vi "SE Update Type.vi"(7 "Name":string, 8 "error in (no error)":errorcluster, 9 "Type":string, 10 "Child Refs":T1[](array[typedef]) format="%.0x", 11 "Type":T2) -> (0 "error out":errorcluster)   [LabVIEW 2015, in "RefMem DMA Custom Device.lvlib"]
uses:
  RefMem DMA Custom Device.lvlib
  Controls/Data Channel Type.ctl
  Program Files (x86)/National Instruments/LabVIEW 2015/vi.lib/NI Veristand/Custom Device API/Custom Device Item Ref.ctl
  Program Files (x86)/National Instruments/LabVIEW 2015/vi.lib/NI Veristand/Custom Device API/Custom Device Channel Type.ctl
  Program Files (x86)/National Instruments/LabVIEW 2015/vi.lib/NI Veristand/Custom Device API/Set Item Property (U16).vi
  Program Files (x86)/National Instruments/LabVIEW 2015/vi.lib/NI Veristand/Custom Device API/Custom Device API.lvlib
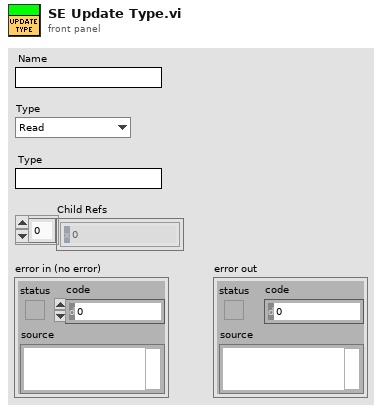
[diagram p1: front panel]
types:
  T1 = typedef "Custom Device API.lvlib/Custom Device Item Ref.ctl" = u64
  T2 = typedef "RefMem DMA Custom Device.lvlib/Data Channel Type.ctl" = enum16{"Read", "Write"}
  T3 = typedef "Custom Device API.lvlib/Custom Device Channel Type.ctl" = enum16{"Input", "Output"}
  T4 = typedef "Custom Device API.lvlib/Custom Device Item Info.ctl" = cluster{"Name":string, "Is Channel":bool, "GUID":string, "Is Waveform":bool}
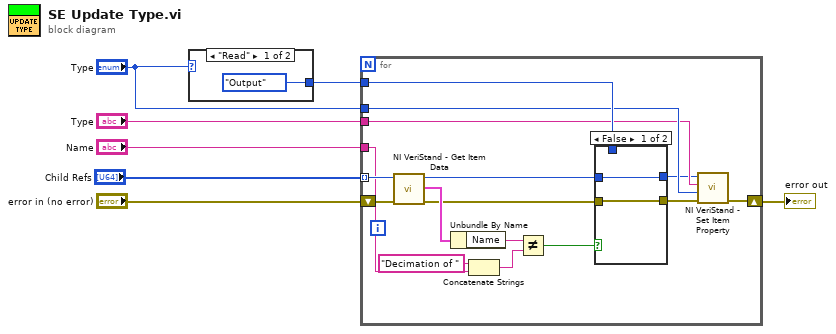
[diagram p0: block diagram]
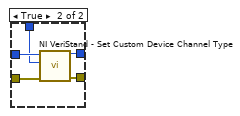
[diagram p2: hidden frame]
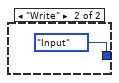
[diagram p3: hidden frame]
diagram:
  n1 = case shown="\"Read\"" "Type" {
    tunnel: [Custom_Device_Channel_Type."Output" ("Type") Custom_Device_Channel_Type."Input" ("Type")] -> w5
    frame "Read" {
    }
    frame "Write" {
    }
  }
  n2 = for {
    shift-right: [w19] -> w2
    shift-left: "error in (no error)" -> [w17]
    tunnel: "Child Refs" -> [w18] mode=indexing
    tunnel: w5 -> [w24]
    tunnel: "Type" -> [w22]
    tunnel: "Type" -> [w21]
    tunnel: "Name" -> [w11]
    n3 = call "NI VeriStand - Get Item Data.vi"("error in (no error)"=w17, "Item Ref in"=w18) -> ("error out"=w15:errorcluster, "Item Info"=w16:T4)  [unwired: 8 out]
    n4 = Unbundle By Name(w16) -> ("Name"=w14:string)
    n5 = Concatenate Strings("Decimation of " ("string"), w11) -> (w12:string)
    n6 = Not Equal?(x=w14, y=w12) -> (x != y?=w10:bool)
    n7 = case shown="False" w10 {
      tunnel: w15 -> [w25 w31]
      tunnel: w18 -> [w26 w30]
      tunnel: w24 -> [_ w29]
      tunnel: [w25 w28] -> w23
      tunnel: [w26 w27] -> w20
      frame False {
      }
      frame True {
        n8 = call "NI VeriStand - Set Custom Device Channel Type.vi"("error in (no error)"=w31, "Type"=w29, "Channel Ref in"=w30) -> ("error out"=w28:errorcluster, "Channel Ref out"=w27:T1)  [unwired: 7 in]
      }
    }
    n9 = call-poly "NI VeriStand - Set Item Property.vi"("error in (no error)"=w23, "Value"=w22, "Property Name"=w21, "Item Ref in"=w20) -> ("error out"=w19:errorcluster)  [unwired: 5 in, 2 out]
  }
  "error out" <- w2
